vi "Test Set Cell Value 2D Array Integer.vi"(11 "Test Case In":refnum<class "Test Open Xml.lvclass">) -> (0 "error out":errorcluster, 3 "Test Case Out":refnum<class "Test Open Xml.lvclass">)   [LabVIEW 2020, in "Test Open Xml.lvclass"]
uses:
  Test Open Xml.lvclass
  <vilib>/Astemes/LUnit/Test Case.lvclass
  Source/Open Xml.lvlib
  7676719e-bc89-419e-861d-f2df32411ec7.vi
  f76079c9-ef62-41ac-a871-70fbb9772100.vi
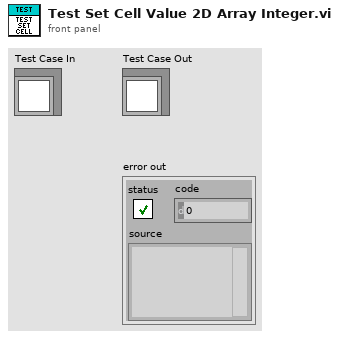
[diagram p1: front panel]
types:
  T1 = typedef "Open Xml.lvlib/Cell DataType.ctl" = enum16{"Void", "Boolean", "Number", "Error", "SharedString", "String", "InlineString", "Date"}
  T2 = cluster{"Number":dbl, "String":string, "Boolean":bool, "Time Stamp":timestamp, "Error":errorcluster}[][]
  T3 = enum16{"Void", "Boolean", "Number", "Error", "SharedString", "String", "InlineString", "Date"}
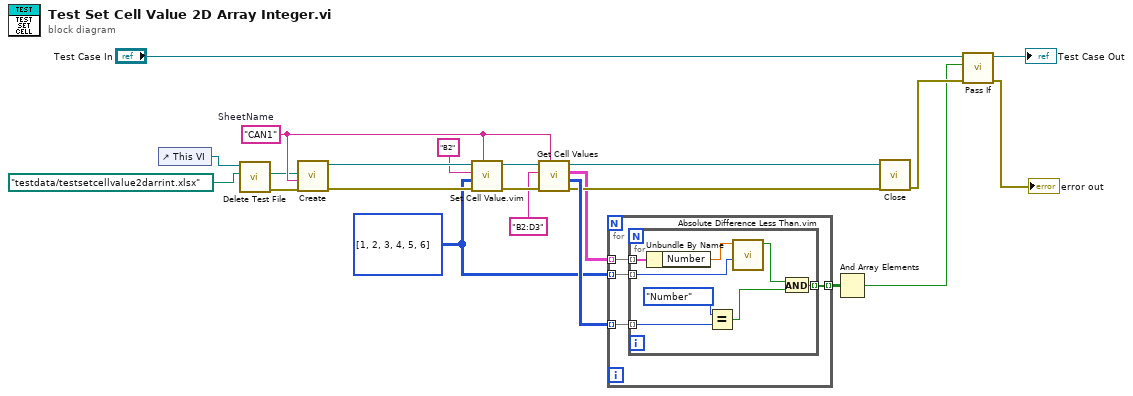
[diagram p0: block diagram]
diagram:
  w4 = i32[][] [[1, 2, 3], [4, 5, 6]]
  w15 = "CAN1"  # SheetName
  n1 = control-ref of="This VI"() -> (w14:refnum<vi>)
  n2 = call "Delete Test File.vi"("name or relative path"=path "testdata/testsetcellvalue2darrint.xlsx", "VI in"=w14) -> ("error out"=w12:errorcluster, "deleted path"=w11:path)  [unwired: 8 in]
  n3 = call "Create.vi"("error in"=w12, "SheetName"=w15, "Path"=w11) -> ("error out"=w18:errorcluster, "SpreadsheetDoc"=w19:refnum<k24>)  [unwired: 7 in]
  n4 = call "Set Cell Value.vim"("Sheet Name"=w15, "error in"=w18, "Value"=w4, "Cell Address"="B2", "SpreadsheetDoc in"=w19) -> ("error out"=w10:errorcluster, "SpreadsheetDoc out"=w9:refnum<k24>)  [unwired: 5 in]
  n5 = call "Get Cell Values.vi"("Sheet Name"=w15, "error in"=w10, "Cell Addresses"="B2:D3", "SpreadsheetDoc in"=w9) -> ("error out"=w5:errorcluster, "Types"=w8:T1[][], "Cell Values"=w3:T2, "SpreadsheetDoc out"=w16:refnum<k24>)  [unwired: 4 in]
  n6 = for {
    tunnel: w8 -> [w26] mode=indexing
    tunnel: w4 -> [w25] mode=indexing
    tunnel: w3 -> [w24] mode=indexing
    tunnel: [w23] -> w2 mode=indexing
    n7 = for {
      tunnel: w26 -> [w33] mode=indexing
      tunnel: w25 -> [w29] mode=indexing
      tunnel: w24 -> [w31] mode=indexing
      tunnel: [w27] -> w23 mode=indexing
      n8 = Unbundle By Name(w31) -> ("Number"=w30:dbl)
      n9 = Equal?(x=T3."Number", y=w33) -> (x = y?=w32:bool)
      n10 = call "Absolute Difference Less Than.vim"("Number 2"=w29, "Number 1"=w30) -> ("In Limit"=w28:bool)  [unwired: 9 in]
      n11 = And(x=w28, y=w32) -> (x .and. y?=w27:bool)
    }
  }
  n12 = And Array Elements(Boolean array=w2) -> (logical AND=w1:bool)
  n13 = call "Close.vi"("error in"=w5, "SpreadsheetDoc"=w16) -> ("error out"=w17:errorcluster)  [unwired: 9 in]
  n14 = call <vilib>:"Pass If.vi"("error in (no error)"=w17, "Pass?"=w1, "LUnit Test Case In"="Test Case In") -> ("error out"=→"error out":errorcluster, "LUnit Test Case Out"=→"Test Case Out":refnum<class "Test Open Xml.lvclass">)  [unwired: 7 in]
